vi "3D-StepNumberAnalyse.vi"(7 "布尔":bool, 9 "StepNumber":i32, 10 "Chose Move Segment":string(combo)="Step_1", 11 "VersionParams":string[][](array[string]) caption="所有行") -> (3 "StepNumberParam":string[][](array[string]))   [LabVIEW 2015]
panel:
  out "StepName":string
  out "StepNumber":i32
  out "子字符串之后":string
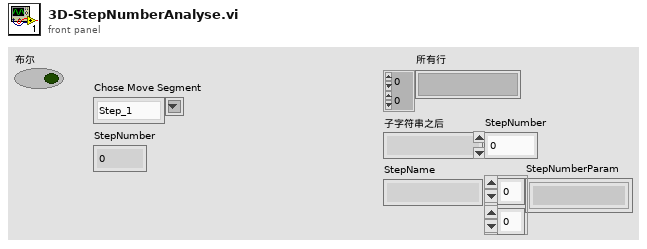
[diagram p1: front panel]
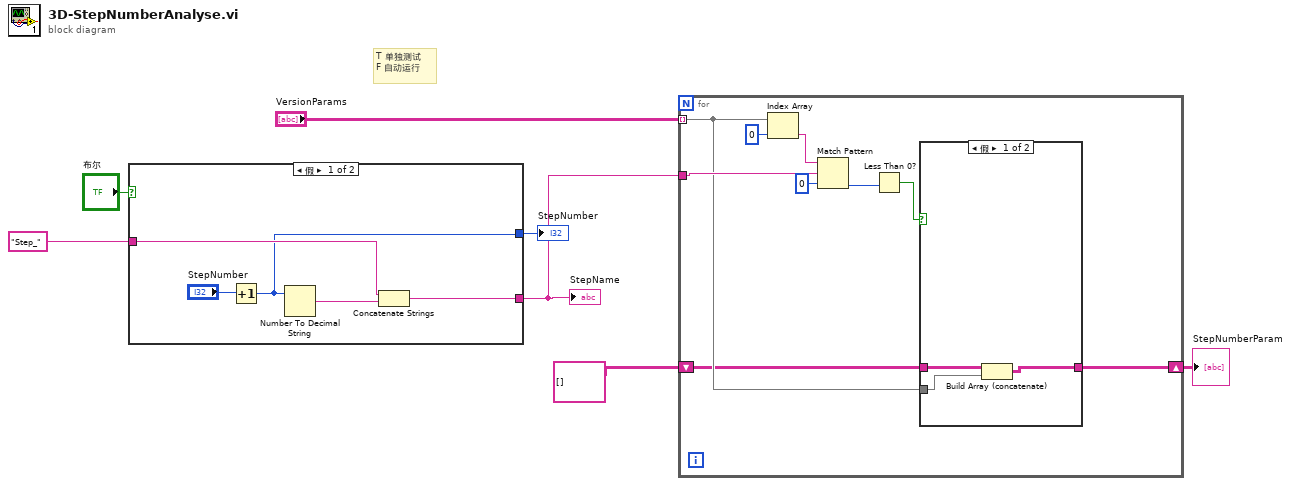
[diagram p0: block diagram]
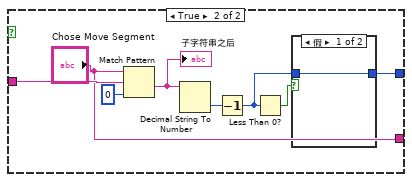
[diagram p3: hidden frame]
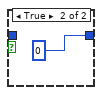
[diagram p4: hidden frame]
diagram:
  # "T 单独测试\nF 自动运行"
  n1 = case shown="假" "布尔" {
    tunnel: "Step_" ("正则表达式") -> [w10 w15]
    tunnel: [w8 w14] -> w6
    tunnel: [w9 "Chose Move Segment"] -> w2
    frame False {
      n2 = Increment(x="StepNumber") -> (x+1=w8:i32)
      n3 = Number To Decimal String(number=w8) -> (decimal integer string=w12:string)  [unwired: 1 in]
      n4 = Concatenate Strings(w10, w12) -> (w9:string)
    }
    frame True {
      n5 = Match Pattern(string="Chose Move Segment", regular expression=w15, offset (0)=0 ("偏移量(0)")) -> (after substring=w19:string)  [unwired: 3 out]
      "子字符串之后" <- w19
      n6 = Decimal String To Number(string=w19) -> (number=w18:i32)  [unwired: 2 in, 1 out]
      n7 = Decrement(x=w18) -> (x-1=w16:i32)
      n8 = Less Than 0?(x=w16) -> (x < 0?=w17:bool)
      n9 = case shown="假" w17 {
        tunnel: [w21 0] -> w14
        tunnel: w16 -> [w21 _]
        frame False {
        }
        frame True {
        }
      }
    }
  }
  "StepNumber" <- w6
  "StepName" <- w2
  n10 = for {
    tunnel: "VersionParams" -> [w25] mode=indexing
    shift-right: [w23] -> w1
    shift-left: string[][] [] -> [w24]
    tunnel: w2 -> [w29]
    n11 = Index Array(array=w25, index=0 ("索引")) -> (element=w30:string)
    n12 = Match Pattern(string=w30, regular expression=w29, offset (0)=0 ("偏移量(0)")) -> (offset past match=w27:i32)  [unwired: 3 out]
    n13 = Less Than 0?(x=w27) -> (x < 0?=w26:bool)
    n14 = case shown="假" w26 {
      tunnel: w25 -> [w33 _]
      tunnel: w24 -> [w34 w35]
      tunnel: [w32 w35] -> w23
      frame False {
        n15 = Build Array (concatenate)(w34, w33) -> (w32:string[][])
      }
      frame True {
      }
    }
  }
  "StepNumberParam" <- w1
